vi "response header.vi"(8 "error in":errorcluster, 10 "Content-Length":i32, 11 "Content String":string) -> (0 "error out":errorcluster, 3 "response string":string)   [LabVIEW 2014]
doc: "Prepends an XML-RPC response header to response message contents"
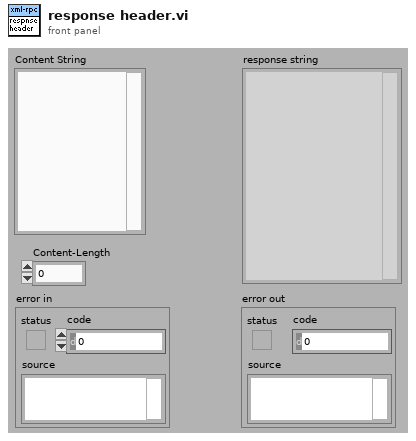
[diagram p1: front panel]
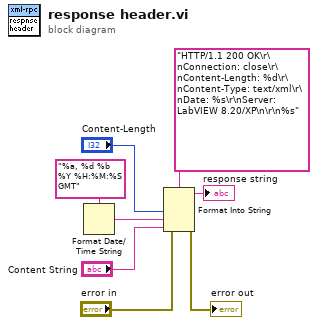
[diagram p0: block diagram]
diagram:
  n1 = Format Date/Time String(time format string (%c)="%a, %d %b %Y %H:%M:%S GMT") -> (date/time string=w7:string)  [unwired: 2 in]
  n2 = Format Into String(format string="HTTP/1.1 200 OK\r\nConnection: close\r\nContent-Length: %d\r\nContent-Type: text/xml\r\nDate: %s\r\nServer: LabVIEW 8.20/XP\n\r\n%s", error in="error in", "Content-Length", w7, "Content String") -> (resulting string=→"response string":string, error out=→"error out":errorcluster)  [unwired: 1 in]
